vi "Record and Save.vi"(8 "Save":bool, 9 "Record":bool, 11 "Inputs":T1={"Slider 1"=0.2727272727272728, "Slider 2"=0.25252525252525265}) -> ()   [LabVIEW 2012]
uses:
  Downloads/Team 1736 Autoflex v1.1 %28Fixed%29 (1)/Joystick Event.ctl
panel:
  out "Info Path":path=path "C:/Users/FRC/Desktop/Autoflex/00.txt"
  out "File Path":path=path "C:/Users/FRC/Desktop/Autoflex/00.autoflex"
  out "Joystick Event":cluster{"Timestamp":u32, "Input":T1}={"Timestamp"=0, "Input"={"Slider 1"=0.2727272727272728, "Slider 2"=0.25252525252525265}}
  out "Timestamp":u32
  out "Joystick Event Array":cluster{"Timestamp":u32, "Input":T1}[](array[cluster])=[{"Timestamp"=0, "Input"={"Slider 1"=0.2727272727272728, "Slider 2"=0.25252525252525265}}]
  out "Array size":i32=1
  out "Last Played Index":i32
  out "Retrieve Index":i32
  out "Start Time":u32=30309169
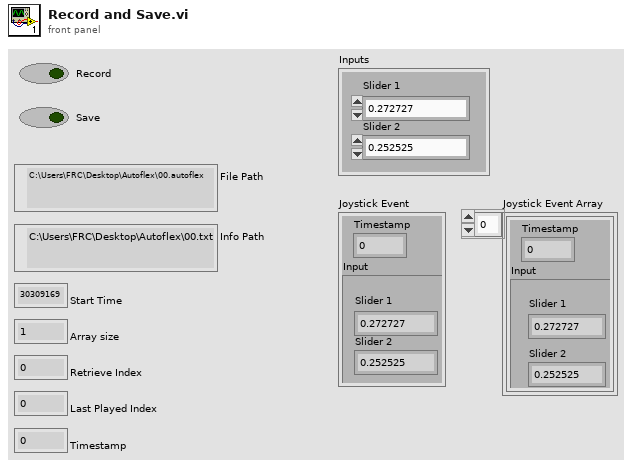
[diagram p1: front panel]
types:
  T1 = typedef "Joystick Event.ctl" = cluster{"Slider 1":dbl, "Slider 2":dbl}
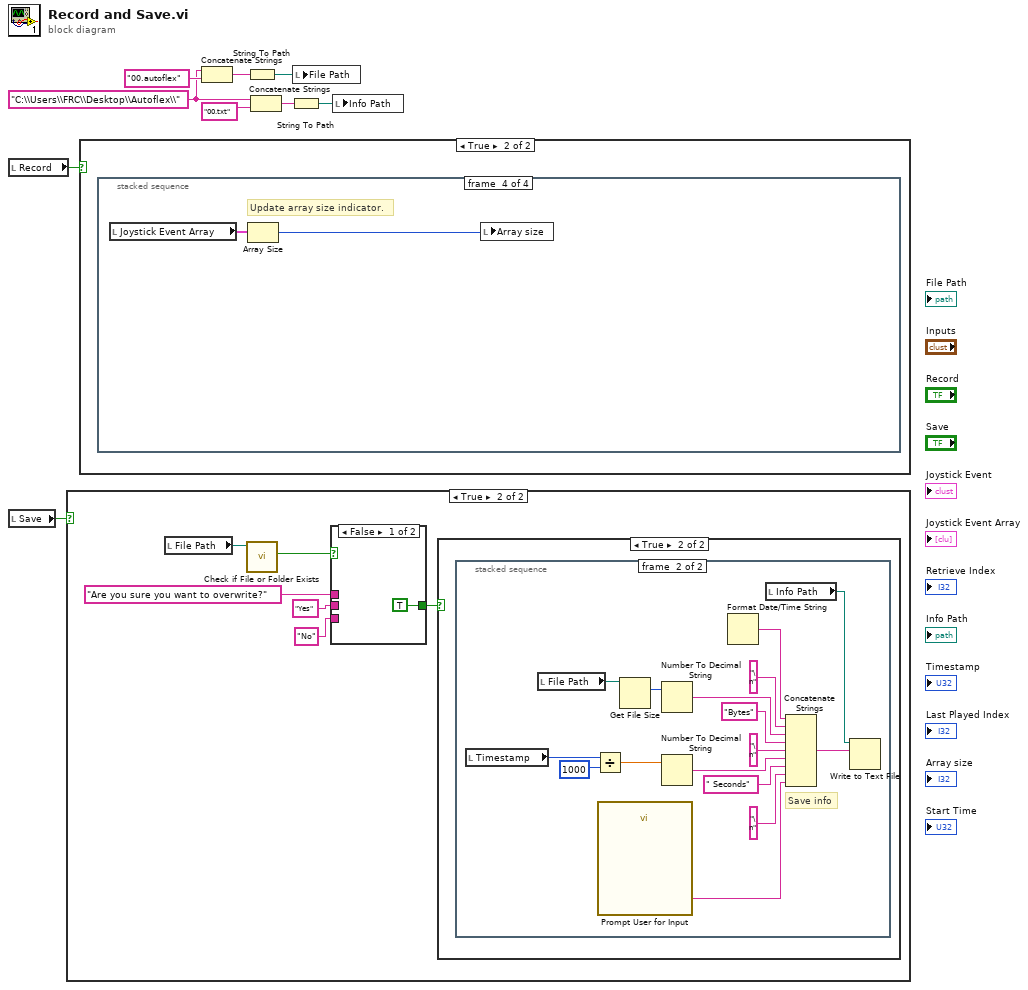
[diagram p0: block diagram]
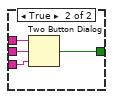
[diagram p3: hidden frame]
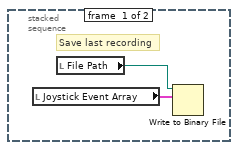
[diagram p5: hidden frame]
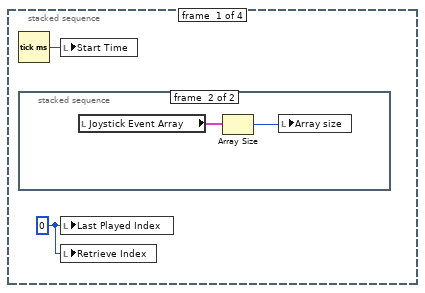
[diagram p7: hidden frame]
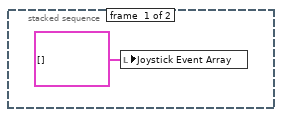
[diagram p8: hidden frame]
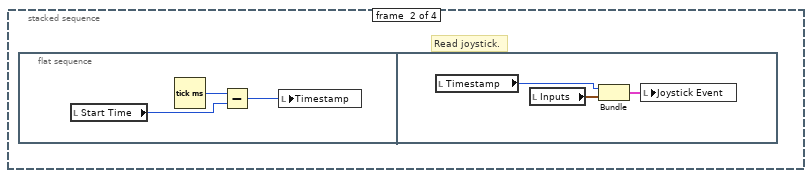
[diagram p9: hidden frame]
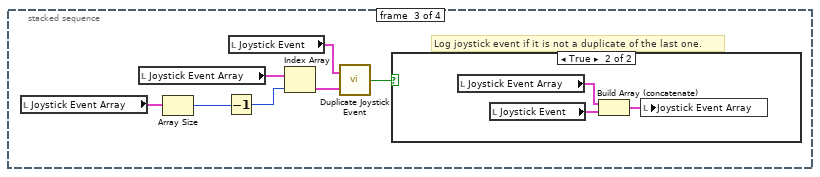
[diagram p10: hidden frame]
diagram:
  w1 = "C:\\Users\\FRC\\Desktop\\Autoflex\\" ("string")
  n1 = local read "Record"() -> (w9:bool)
  n2 = local read "Save"() -> (w8:bool)
  n3 = case shown="True" w8 {
    frame False {
    }
    frame True {
      n4 = local read "File Path"() -> (w13:path)
      n5 = call <vilib>:"Check if File or Folder Exists.vi"("path"=w13) -> ("file or folder exists?"=w14:bool)  [unwired: 1 in, 9 out]
      n6 = case shown="False" w14 {
        tunnel: [TRUE ("T button?") w20] -> w15
        tunnel: "Are you sure you want to overwrite?" ("message") -> [_ w19]
        tunnel: "Yes" ("T button name (\"OK\")") -> [_ w18]
        tunnel: "No" ("T button name (\"OK\")") -> [_ w17]
        frame False {
        }
        frame True {
          n7 = Two Button Dialog(message=w19, 1:w17, 2:w18) -> (T button?=w20:bool)
        }
      }
      n8 = case shown="True" w15 {
        frame False {
        }
        frame True {
          n9 = stacked-sequence {
            frame #0 {
              # "Save last recording"
              n10 = local read "Joystick Event Array"() -> (w21:cluster{"Timestamp":u32, "Input":T1}[])
              n11 = local read "File Path"() -> (w22:path)
              n12 = Write to Binary File(file (use dialog)=w22, data=w21) -> ()  [unwired: 1 in, 6 out]
            }
            frame #1 {
              # "Save info"
              n13 = local read "Timestamp"() -> (w29:u32)
              n14 = local read "File Path"() -> (w38:path)
              n15 = Divide(x=w29, y=u32 1000) -> (x/y=w26:dbl)
              n16 = call "Prompt User for Input"() -> ("Comments"=w24:string)  [unwired: 2 in, 17 out]
              n17 = Get File Size(file=w38) -> (size (in bytes)=w37:i64)  [unwired: 1 in, 2 out]
              n18 = Number To Decimal String(number=w37) -> (decimal integer string=w32:string)  [unwired: 1 out]
              n19 = Number To Decimal String(number=w26) -> (decimal integer string=w27:string)  [unwired: 1 out]
              n20 = Format Date/Time String() -> (date/time string=w34:string)  [unwired: 3 out]
              n21 = local read "Info Path"() -> (w36:path)
              n22 = Concatenate Strings(w34, "\n" ("string"), w32, "Bytes" ("string"), "\n" ("string"), w27, " Seconds" ("string"), "\n" ("string"), w24) -> (w35:string)
              n23 = Write to Text File(file (use dialog)=w36, text=w35) -> ()  [unwired: 1 in, 4 out]
            }
          }
        }
      }
    }
  }
  n24 = case shown="True" w9 {
    frame False {
    }
    frame True {
      n25 = stacked-sequence {
        frame #0 {
          w39 = 0 ("index")
          n26 = Tick Count (ms)() -> (millisecond timer value=w40:u32)
          n27 = stacked-sequence {
            frame #0 {
              n28 = local write "Joystick Event Array"(cluster{"Timestamp":u32, "Input":T1}[] [] ("Joystick Event Array")) -> ()
            }
            frame #1 {
              n29 = local read "Joystick Event Array"() -> (w42:cluster{"Timestamp":u32, "Input":T1}[])
              n30 = Array Size(array=w42) -> (size(s)=w43:i32)
              n31 = local write "Array size"(w43) -> ()
            }
          }
          n32 = local write "Start Time"(w40) -> ()
          n33 = local write "Last Played Index"(w39) -> ()
          n34 = local write "Retrieve Index"(w39) -> ()
        }
        frame #1 {
          # "Read joystick."
          n35 = flat-sequence {
            frame #0 {
              n36 = local read "Start Time"() -> (w45:u32)
              n37 = Tick Count (ms)() -> (millisecond timer value=w44:u32)
              n38 = Subtract(x=w44, y=w45) -> (x-y=w46:u32)
              n39 = local write "Timestamp"(w46) -> ()
            }
            frame #1 {
              n40 = local read "Timestamp"() -> (w48:u32)
              n41 = local read "Inputs"() -> (w47:T1)
              n42 = Bundle("Timestamp"=w48, "Inputs"=w47) -> (w49:cluster{"Timestamp":u32, "Inputs":T1})  [unwired: 1 out]
              n43 = local write "Joystick Event"(w49) -> ()
            }
          }
        }
        frame #2 {
          # "Log joystick event if it is not a duplicate of the last one."
          n44 = local read "Joystick Event Array"() -> (w54:cluster{"Timestamp":u32, "Input":T1}[])
          n45 = local read "Joystick Event Array"() -> (w53:cluster{"Timestamp":u32, "Input":T1}[])
          n46 = Array Size(array=w54) -> (size(s)=w56:i32)
          n47 = Decrement(x=w56) -> (x-1=w55:i32)
          n48 = local read "Joystick Event"() -> (w51:cluster{"Timestamp":u32, "Input":T1})
          n49 = Index Array(array=w53, index=w55) -> (element=w52:cluster{"Timestamp":u32, "Input":T1})
          n50 = call "Duplicate Joystick Event.vi"("Joystick Event 2"=w52, "Joystick Event 1"=w51) -> ("Duplicate"=w50:bool)
          n51 = case shown="True" w50 {
            frame False {
            }
            frame True {
              n52 = local read "Joystick Event Array"() -> (w57:cluster{"Timestamp":u32, "Input":T1}[])
              n53 = local read "Joystick Event"() -> (w59:cluster{"Timestamp":u32, "Input":T1})
              n54 = Build Array (concatenate)(w57, w59) -> (w58:cluster{"Timestamp":u32, "Input":T1}[])
              n55 = local write "Joystick Event Array"(w58) -> ()
            }
          }
        }
        frame #3 {
          # "Update array size indicator."
          n56 = local read "Joystick Event Array"() -> (w60:cluster{"Timestamp":u32, "Input":T1}[])
          n57 = Array Size(array=w60) -> (size(s)=w61:i32)
          n58 = local write "Array size"(w61) -> ()
        }
      }
    }
  }
  n59 = Concatenate Strings(w1, "00.autoflex" ("string")) -> (w4:string)
  n60 = String To Path(string=w4) -> (path=w6:path)
  n61 = Concatenate Strings(w1, "00.txt" ("string")) -> (w3:string)
  n62 = String To Path(string=w3) -> (path=w5:path)
  n63 = local write "File Path"(w6) -> ()
  n64 = local write "Info Path"(w5) -> ()
